vi "3D Obstacles.vi"(1 "Obstacles (n x 2 array of pts)":cluster{dbl, dbl}[][](array[cluster]), 2 "Height":dbl, 3 "Name":string) -> (0 "Scene:New Object":refnum<vi>)   [LabVIEW 2011]
uses:
  3D Point.ctl
  <vilib>/Utility/miscctls.llb/LVRGBAColorTypeDef.ctl
  <vilib>/picture/3D Picture Control/NI_3D Picture Control.lvlib
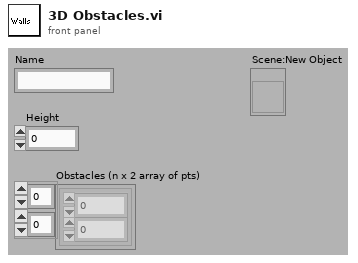
[diagram p1: front panel]
types:
  T1 = enum16{"Overall", "Per Primitive", "Per Vertex", "Binding Off"}
  T2 = typedef "LVRGBAColorTypeDef.ctl" = cluster{"Red":sgl, "Green":sgl, "Blue":sgl, "Alpha":sgl}
  T3 = enum16{"Points", "Lines", "Line Strip", "Line Loop", "Triangles", "Triangle Strip", "Triangle Fan", "Quads", "Quad Strip", "Polygon"}
  T4 = typedef "3D Point.ctl" = cluster{"X":dbl, "Y":dbl, "Z":dbl}
  T5 = typedef "2D Point.ctl" = cluster{"X":dbl, "Y":dbl}
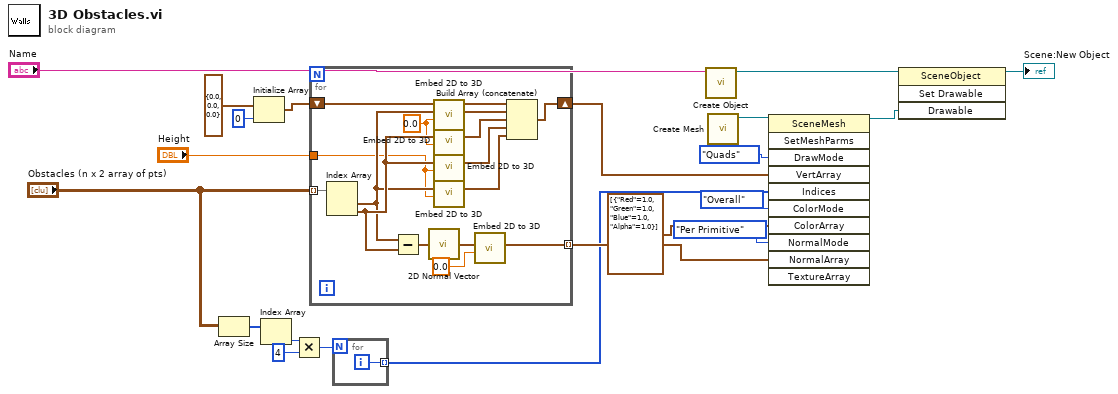
[diagram p0: block diagram]
diagram:
  n1 = Array Size(array="Obstacles (n x 2 array of pts)") -> (size(s)=w9:i32[])
  n2 = Initialize Array(T4 {"X"=0.0, "Y"=0.0, "Z"=0.0} ("3D Point"), 0 ("dimension size")) -> (w1:T4[])
  n3 = Index Array(array=w9) -> (element=w11:i32)  [unwired: 1 in]
  n4 = Multiply(x=w11, y=4) -> (x*y=w13:i32)
  n5 = for {
    tunnel: "Obstacles (n x 2 array of pts)" -> [w36] mode=indexing
    tunnel: [w34] -> w18 mode=indexing
    shift-right: [w24] -> w8
    shift-left: w1 -> [w32]
    tunnel: "Height" -> [w22]
    w23 = 0.0 ("Z")
    n6 = Index Array(array=w36) -> (element #1=w29:cluster{dbl, dbl}, element #2=w30:cluster{dbl, dbl})  [unwired: 2 in]
    n7 = Subtract(x=w29, y=w30) -> (x-y=w35:cluster{dbl, dbl})
    n8 = call "2D Normal Vector.vi"("2D Vector"=w35) -> ("2D Normal"=w31:T5)  [unwired: 4 out]
    n9 = call "Embed 2D to 3D.vi"("Z"=w23, "2D Point"=w29) -> ("3D Point"=w28:T4)  [unwired: 7 out]
    n10 = call "Embed 2D to 3D.vi"("Z"=w23, "2D Point"=w30) -> ("3D Point"=w27:T4)  [unwired: 7 out]
    n11 = call "Embed 2D to 3D.vi"("Z"=w22, "2D Point"=w30) -> ("3D Point"=w26:T4)  [unwired: 7 out]
    n12 = call "Embed 2D to 3D.vi"("Z"=w22, "2D Point"=w29) -> ("3D Point"=w25:T4)  [unwired: 7 out]
    n13 = call "Embed 2D to 3D.vi"("Z"=0.0, "2D Point"=w31) -> ("3D Point"=w34:T4)  [unwired: 7 out]
    n14 = Build Array (concatenate)(w32, w28, w27, w26, w25) -> (w24:T4[])
  }
  n15 = for {
    N: w13 -> [_]
    tunnel: [w37] -> w14 mode=indexing
    i -> [w37]
  }
  n16 = call <vilib>:"Create Object.vi"("Name"="Name") -> ("Scene:New Object"=w19:refnum<vi>)  [unwired: 1 in, 9 out]
  n17 = call <vilib>:"Create Mesh.vi"() -> ("New Mesh Refnum"=w6:refnum<vi>)  [unwired: 1 in, 10 out]
  n18 = invoke class="SceneMesh" method="SetMeshParms"(reference=w6, "DrawMode"=T3."Quads" ("Draw Mode"), "VertArray"=w8, "Indices"=w14, "ColorMode"=T1."Overall" ("Color Binding Mode"), "ColorArray"=T2[] [{"Red"=1.0, "Green"=1.0, "Blue"=1.0, "Alpha"=1.0}] ("Color Array"), "NormalMode"=T1."Per Primitive" ("Normal Binding Mode"), "NormalArray"=w18) -> (reference out=w20:refnum<vi>)  [unwired: 3 in, 10 out]
  n19 = invoke class="SceneObject" method="Set Drawable"(reference=w19, "Drawable"=w20) -> (reference out=→"Scene:New Object":refnum<vi>)  [unwired: 2 in, 3 out]
